vi "Get Element References by Tag Name.vi"(6 "required (F)":bool, 8 "error in":errorcluster, 10 "tag name":string, 11 "node in":refnum<k20>) -> (0 "error out":errorcluster, 3 "array of elements":refnum<k20>[](array[refnum]))   [LabVIEW 2020, in "MIL-STD 1553 Import.lvlib"]
uses:
  MIL-STD 1553 Import.lvlib
  <resource>/objmgr/DOMUserDefRef.rc
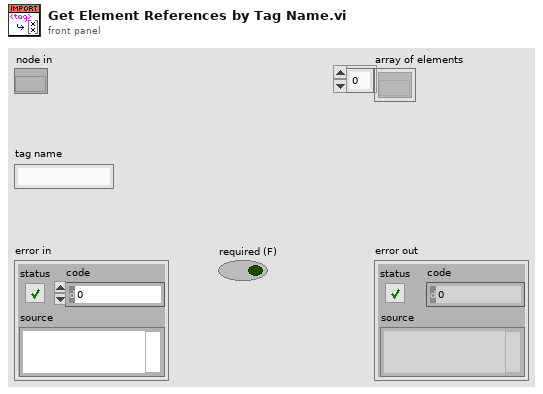
[diagram p1: front panel]
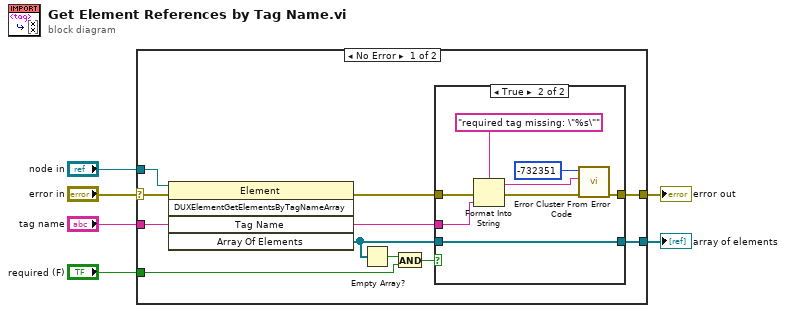
[diagram p0: block diagram]
diagram:
  n1 = case shown="No Error" "error in" {
    selector: "error in" -> [w15 w27]
    tunnel: [w13 w27] -> w5
    tunnel: [w14 _] -> w4
    tunnel: "node in" -> [w16 _]
    tunnel: "tag name" -> [w11 _]
    tunnel: "required (F)" -> [w8 _]
    frame No Error {
      n2 = invoke class="Element" method="DUXElementGetElementsByTagNameArray"(reference=w16, error in=w15, "Tag Name"=w11) -> (error out=w12:errorcluster, "Array Of Elements"=w9:refnum<k20>[])  [unwired: 2 in, 3 out]
      n3 = Empty Array?(array=w9) -> (empty?=w10:bool)
      n4 = And(x=w10, y=w8) -> (x .and. y?=w7:bool)
      n5 = case shown="True" w7 {
        tunnel: [w18 w19] -> w14
        tunnel: w9 -> [w18 w19]
        tunnel: [w17 w21] -> w13
        tunnel: w12 -> [w17 w23]
        tunnel: w11 -> [_ w20]
        frame False {
        }
        frame True {
          n6 = Format Into String(format string="required tag missing: \"%s\"", error in=w23, w20) -> (resulting string=w26:string, error out=w22:errorcluster)  [unwired: 1 in]
          n7 = call <vilib>:"Error Cluster From Error Code.vi"("error in (no error)"=w22, "error message (\"\")"=w26, "error code (0)"=-732351) -> ("error out"=w21:errorcluster)  [unwired: 6 in]
        }
      }
    }
    frame Error {
    }
  }
  "error out" <- w5
  "array of elements" <- w4
